vi "GetAxisFromProject.vi"(8 "error in (no error)":errorcluster, 11 "Path":path) -> (0 "error out":errorcluster, 1 "Axis Array":string[](array[string]), 2 "Coordinate System Array":string[](array[string]))   [LabVIEW 2017, in "ProjectUtilities.lvlib"]
uses:
  ProjectUtilities.lvlib
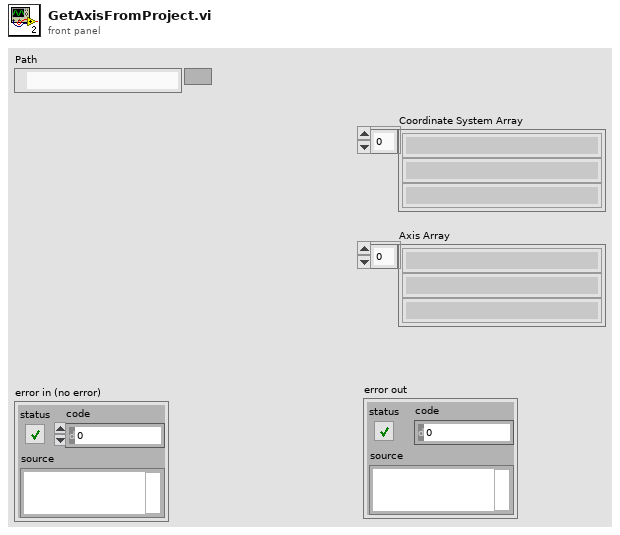
[diagram p1: front panel]
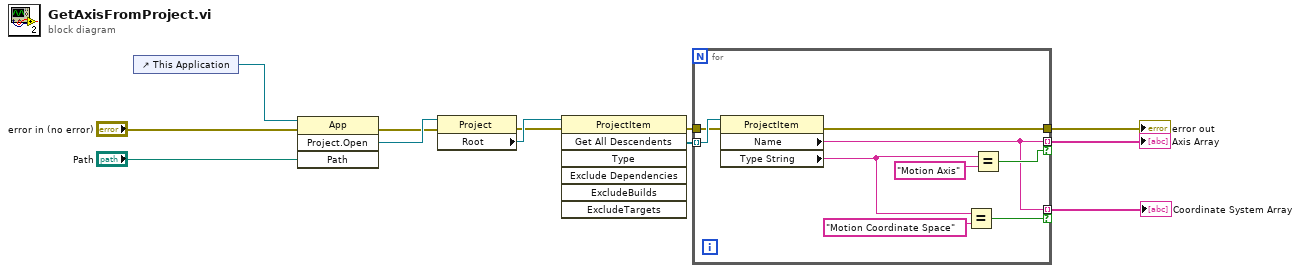
[diagram p0: block diagram]
diagram:
  n1 = control-ref of="This Application"() -> (w12:refnum<vi>)
  n2 = invoke class="App" method="Project.Open"(reference=w12, error in="error in (no error)", "Path"="Path") -> (error out=w6:errorcluster, "Project:Open"=w10:refnum<vi>)  [unwired: 1 in, 2 out]
  n3 = property class="Project"(reference=w10, error in=w6) -> (error out=w5:errorcluster, "Root"=w9:refnum<vi>)  [unwired: 1 out]
  n4 = invoke class="ProjectItem" method="Get All Descendents"(reference=w9, error in=w5) -> (error out=w4:errorcluster, "All Descendents"=w8:refnum<vi>[])  [unwired: 5 in, 5 out]
  n5 = for {
    tunnel: w8 -> [w21] mode=indexing
    tunnel: [w17] -> w7 mode=indexing if=w18
    tunnel: w4 -> [w19]
    tunnel: [w17] -> w3 mode=indexing if=w15
    tunnel: [w13] -> w1
    n6 = property class="ProjectItem"(reference=w21, error in=w19) -> (error out=w13:errorcluster, "Name"=w17:string, "Type String"=w16:string)  [unwired: 1 out]
    n7 = Equal?(x=w16, y="Motion Coordinate Space") -> (x = y?=w15:bool)
    n8 = Equal?(x=w16, y="Motion Axis") -> (x = y?=w18:bool)
  }
  "Axis Array" <- w7
  "Coordinate System Array" <- w3
  "error out" <- w1
